vi "PicoScope6000SetDataBuffers.vi"(5 "enabled array":i16[](array[numeric]), 7 "Buffer and Transfer Settings":T3 {"Down-Sample Mode" items=["None", "Aggregate", "Decimate", "Average"]; "Down Sample Ratio" step=1; "Samples" format="%_6p"}, 8 "error in (no error)":errorcluster, 9 "Device Info":T1, 10 "Data Pointers In":T2, 11 "handle in":i16) -> (0 "error out":errorcluster, 3 "handle out":i16)   [LabVIEW 2009]
doc: "Calls SetDataBuffers, and assigns Pico buffers"
uses:
  ps6000.dll
  shared/PicoBuffers.ctl
  shared/Buffer and Transfer Settings.ctl
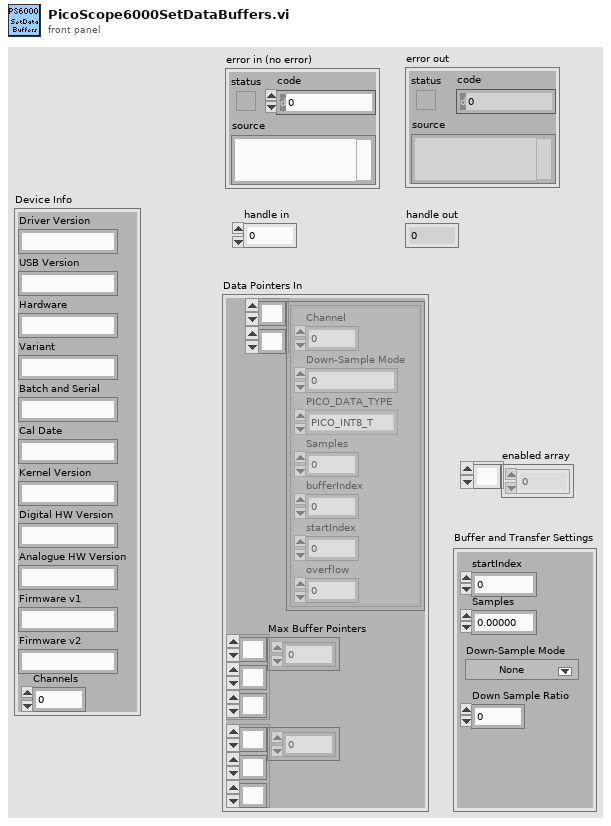
[diagram p1: front panel]
types:
  T1 = cluster{"Driver Version":string, "USB Version":string, "Hardware":string, "Variant":string, "Batch and Serial":string, "Cal Date":string, "Kernel Version":string, "Digital HW Version":string, "Analogue HW Version":string, "Firmware v1":string, "Firmware v2":string, "Channels":i16}
  T2 = typedef "PicoBuffers.ctl" = cluster{"Max Buffer Pointers":u64[][][], "Min Buffer Pointers":u64[][][], "StreamingDataInfo":cluster{"Channel":u32, "Down-Sample Mode":u32, "PICO_DATA_TYPE":enum32{"PICO_INT8_T", "PICO_INT16_T", "PICO_INT32_T", "PICO_UINT32_T", "PICO_INT64_T", ""}, "Samples":i32, "bufferIndex":u64, "startIndex":i32, "overflow":i16}[][]}
  T3 = typedef "Buffer and Transfer Settings.ctl" = cluster{"startIndex":u64, "Samples":u64, "Down Sample Ratio":u64, "Down-Sample Mode":u32}
  T4 = cluster{"status":bool, "code":u32, "source":string}
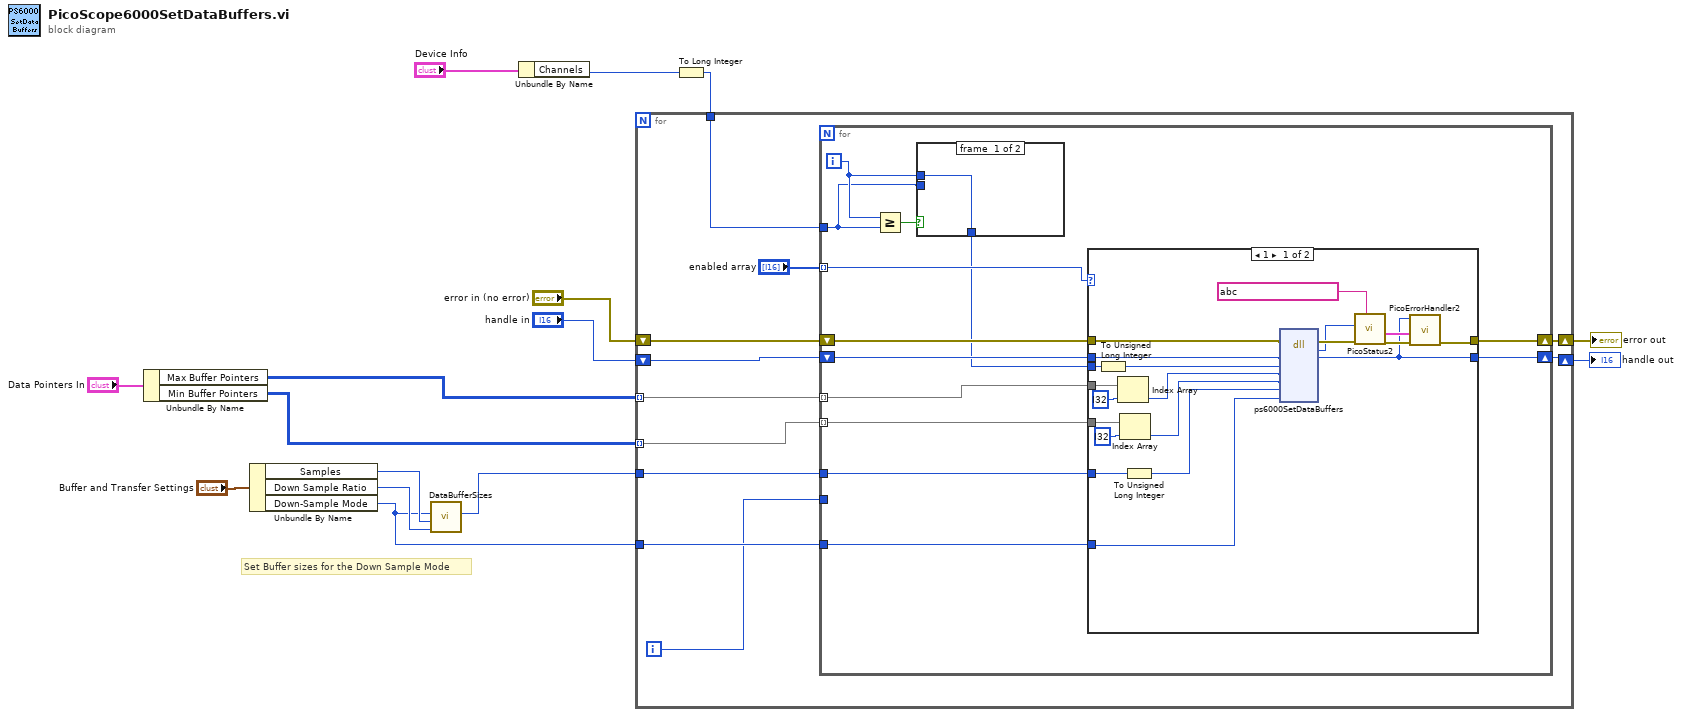
[diagram p0: block diagram]
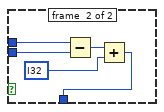
[diagram p2: hidden frame]
diagram:
  # "Set Buffer sizes for the Down Sample Mode"
  n1 = Unbundle By Name("Data Pointers In") -> ("Max Buffer Pointers"=w5:u64[][][], "Min Buffer Pointers"=w4:u64[][][])
  n2 = Unbundle By Name("Buffer and Transfer Settings") -> ("Samples"=w7:u64, "Down Sample Ratio"=w8:u64, "Down-Sample Mode"=w6:u32)
  n3 = call "DataBufferSizes.vi"("Down Sample Ratio"=w8, "Number of Samples"=w7, "Down-Sample Mode"=w6) -> ("Max Buffer Size"=w9:i32)  [unwired: 7 in, 1 out]
  n4 = Unbundle By Name("Device Info") -> ("Channels"=w2:i16)
  n5 = To Long Integer(number=w2) -> (32bit integer=w3:i32)
  n6 = for {
    tunnel: w9 -> [w22]
    tunnel: w6 -> [w21]
    tunnel: w5 -> [w20] mode=indexing
    tunnel: w4 -> [w19] mode=indexing
    shift-right: [w26] -> w14
    shift-left: "error in (no error)" -> [w24]
    shift-right: [w25] -> w13
    shift-left: "handle in" -> [w23]
    tunnel: w3 -> [w16]
    i -> [w17]
    n7 = for {
      tunnel: w21 -> [w39]
      tunnel: w22 -> [w36]
      tunnel: "enabled array" -> [w28] mode=indexing
      tunnel: w20 -> [w35] mode=indexing
      shift-right: [w34] -> w26
      shift-left: w24 -> [w38]
      tunnel: w19 -> [w33] mode=indexing
      shift-right: [w32] -> w25
      shift-left: w23 -> [w37]
      tunnel: w17 -> [_]
      tunnel: w16 -> [w29]
      i -> [w30]
      n8 = Greater Or Equal?(x=w30, y=w29) -> (x >= y?=w31:bool)
      n9 = case shown="True" w31 {
        tunnel: [w40 w44] -> w27
        tunnel: w29 -> [_ w43]
        tunnel: w30 -> [w40 w42]
        frame #0 {
        }
        frame #1 {
          n10 = Subtract(x=w42, y=w43) -> (x-y=w41:i32)
          n11 = Add(x=w41, y=i32 ?) -> (x+y=w44:i32)
        }
      }
      n12 = case shown="1" w28 {
        tunnel: w27 -> [w64 _]
        tunnel: w38 -> [w59 w67]
        tunnel: w37 -> [w58 w66]
        tunnel: w39 -> [w54 _]
        tunnel: [w48 w67] -> w34
        tunnel: [w47 w66] -> w32
        tunnel: w36 -> [w65 _]
        tunnel: w35 -> [w62 _]
        tunnel: w33 -> [w60 _]
        frame #0 {
          n13 = To Unsigned Long Integer(number=w64) -> (unsigned 32bit integer=w57:u32)
          n14 = Index Array(array=w62, index=i32 ?) -> (element=w56:u64)
          n15 = Index Array(array=w60, index=i32 ?) -> (element=w55:u64)
          n16 = To Unsigned Long Integer(number=w65) -> (unsigned 32bit integer=w53:u32)
          n17 = dll-call lib="PS6000.dll" fn="ps6000SetDataBuffers" ("ps3000.dll:_ps3000_open_unit@0")(error in=w59, "handle"=w58, "channel"=w57, "bufferMax"=w56, "bufferMin"=w55, "bufferLth"=w53, "downSampleRatioMode"=w54) -> (error out=w50:errorcluster, "PICO_STATUS"=w49:u32, "handle"=w47:i16)  [unwired: 7 in, 1 out]
          n18 = call "PicoStatus2.vi"("PICO source"=string ? ("source"), "Error in"=w50, "PICO STATUS"=w49) -> ("error out"=w52:errorcluster, "PICO_STATUS out"=w51:T4)  [unwired: 5 in]
          n19 = call "PicoErrorHandler2.vi"("error in (no error)"=w52, "PICO_STATUS in"=w51, "handle In"=w47) -> ("error out"=w48:errorcluster)  [unwired: 8 in]
        }
        frame #1 {
        }
      }
    }
  }
  "error out" <- w14
  "handle out" <- w13
